vi "Set Mode.vi"(8 "error in (no error)":errorcluster, 10 "mode":u8(ring) items=["once", "continous"], 11 "CS++PPG in":refnum<class "CS++PPG.lvclass">) -> (0 "error out":errorcluster, 3 "CS++PPG out":refnum<class "CS++PPG.lvclass">)   [LabVIEW 2016, in "CS++PPG.lvlib" / "CS++PPG.lvclass"]
doc: "This Vi sets the mode of the PPG (0 - single run, 1 - continous)."
uses:
  CS++PPG.lvclass
  CSPP_Core/Classes/CS++ProcessVariables/ProcessVariable/PV.lvclass
  PV-Enum.ctl
  CS++PPG.lvclass/CS++PPG.ctl
  CSPP_Core/Classes/CS++ProcessVariables/ProcessVariable/PV.lvclass/PV.ctl
  CSPP_Core/Classes/CS++ProcessVariables/ProcessVariable/Write Data.vi
  CSPP_Core/Classes/CS++ProcessVariables/ProcessVariable/Write Timestamp.vi
  CSPP_Core/Classes/CS++ProcessVariables/ProcessVariable/Write Quality.vi
  CSPP_Core/Classes/CS++ProcessVariables/ProcessVariable/Write status.vi
  CSPP_Core/Classes/CS++ProcessVariables/PVConnection/PVConnection.lvclass
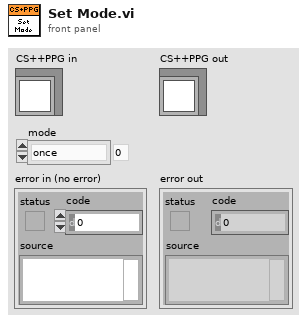
[diagram p1: front panel]
types:
  T1 = typedef "CS++PPG.lvlib/CS++PPG.lvclass/PV-Enum.ctl" = enum16{"Mode", "Trigger"}
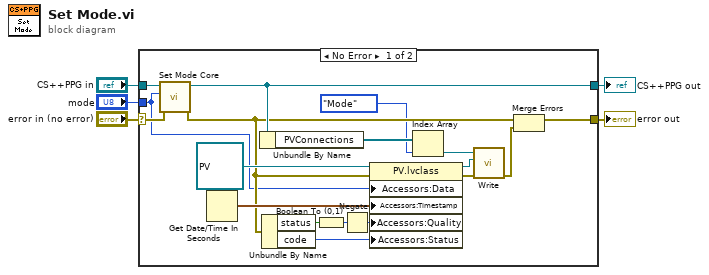
[diagram p0: block diagram]
diagram:
  n1 = case shown="No Error" "error in (no error)" {
    selector: "error in (no error)" -> [w22 w25]
    tunnel: [w9 w25] -> w4
    tunnel: [w11 w24] -> w2
    tunnel: "CS++PPG in" -> [w23 w24]
    tunnel: "mode" -> [w7 _]
    frame No Error {
      n2 = call-dynamic "Set Mode Core.vi"("error in (no error)"=w22, "mode"=w7, "CS++PPG in"=w23) -> ("error out"=w10:errorcluster, "CS++PPG out"=w11:refnum<class "CS++PPG.lvclass">)  [unwired: 7 in]
      n3 = Get Date/Time In Seconds() -> (seconds since 1Jan1904=w21:timestamp)
      n4 = Unbundle By Name(w11) -> ("PVConnections"=w13:refnum<class "PVConnection.lvclass">[])
      n5 = Unbundle By Name(w10) -> ("status"=w16:bool, "code"=w19:i32)
      n6 = Boolean To (0,1)(Boolean=w16) -> (0, 1=w18:i16)
      n7 = Negate(x=w18) -> (-x=w17:i16)
      n8 = property class="PV.lvclass"(reference=refnum<class "PV.lvclass"> refnum ("PV"), error in=w10, "Accessors:Data"=w7, "Accessors:Timestamp"=w21, "Accessors:Quality"=w17, "Accessors:Status"=w19) -> (reference out=w15:refnum<class "PV.lvclass">, error out=w14:errorcluster)
      n9 = Index Array(array=w13, index=PV-Enum."Mode" ("PV-Enum")) -> (element=w12:refnum<class "PVConnection.lvclass">)
      n10 = call "Write.vi"("error in (no error)"=w14, "PV"=w15, "PVConnection in"=w12) -> ("error out"=w8:errorcluster)  [unwired: 7 in, 1 out]
      n11 = Merge Errors(w10, w8) -> (w9:errorcluster)
    }
    frame Error {
    }
  }
  "error out" <- w4
  "CS++PPG out" <- w2
